vi "Result.Build Attribute Result Item.vi"(6 "ForceFail":bool, 7 "Log(F)/Pass(T)":bool, 8 "Error In(Result Error)":errorcluster, 9 "Value":string, 10 "Name":string, 11 "Category":string) -> (0 "Error Out(No Error)":errorcluster, 2 "Fail/Error":bool, 3 "Attribute":T1 {"Status" items=["LOG", "PASS", "FAIL", "ERROR"]})   [LabVIEW 2018]
uses:
  Result.Attribute.ctl
  Result.Measurement and Attribute Item Status.ctl
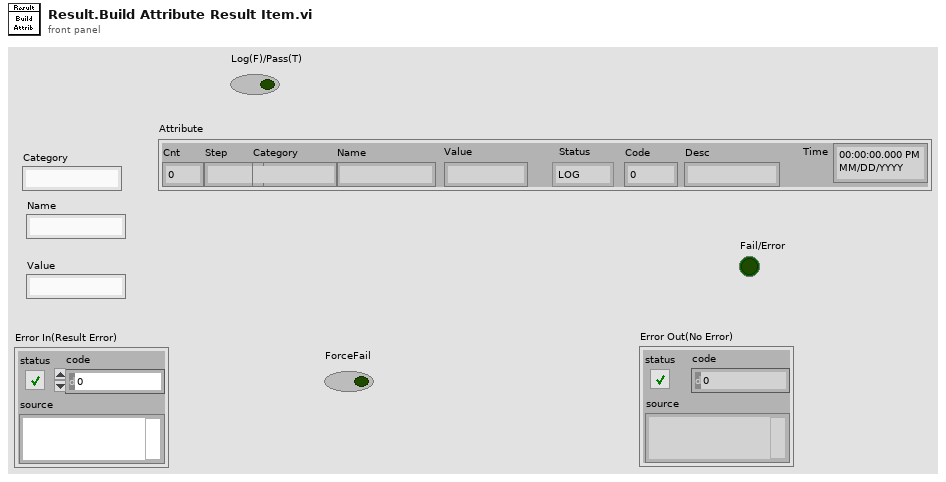
[diagram p1: front panel]
types:
  T1 = typedef "Result.Attribute.ctl" = cluster{"Cnt":i32, "Step":string, "Category":string, "Name":string, "Value":string, "Status":T2, "Code":i32, "Desc":string, "Time":timestamp}
  T2 = typedef "Result.Measurement and Attribute Item Status.ctl" = i32
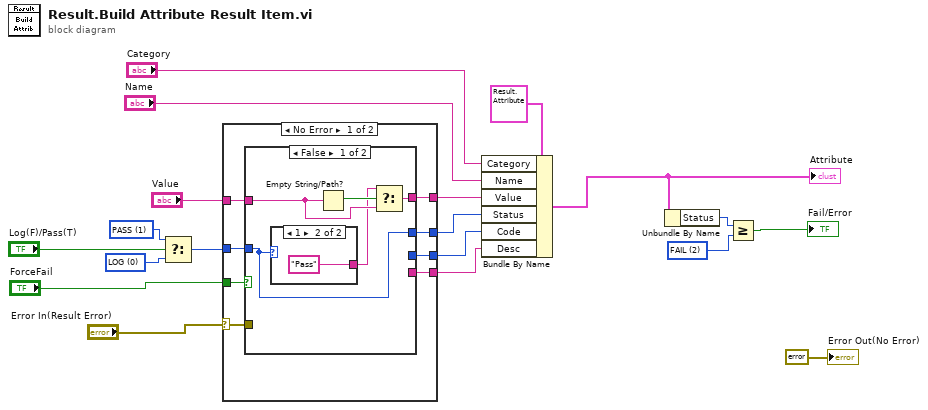
[diagram p0: block diagram]
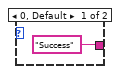
[diagram p2: hidden frame]
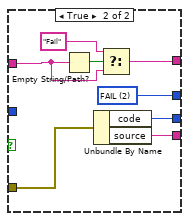
[diagram p3: hidden frame]
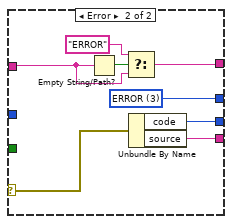
[diagram p4: hidden frame]
diagram:
  w8 = T2 1 items=["LOG", "PASS", "FAIL", "ERROR"] ("Status")
  w7 = T2 0 items=["LOG", "PASS", "FAIL", "ERROR"] ("Status")
  w14 = T2 2 items=["LOG", "PASS", "FAIL", "ERROR"] ("y")
  n1 = Select(t=w8, s="Log(F)/Pass(T)", f=w7) -> (s? t:f=w5:T2)
  n2 = case shown="No Error" "Error In(Result Error)" {
    selector: "Error In(Result Error)" -> [w20 w44]
    tunnel: "ForceFail" -> [w27 _]
    tunnel: [w26 w47] -> w11
    tunnel: [w25 w46] -> w10
    tunnel: [w24 w45] -> w9
    tunnel: w5 -> [w23 _]
    tunnel: "Value" -> [w22 w43]
    tunnel: [w21 w48] -> w2
    frame No Error {
      n3 = case shown="False" w27 {
        tunnel: [w29 w42] -> w26
        tunnel: w20 -> [_ w41]
        tunnel: [_ w40] -> w25
        tunnel: [_ w39] -> w24
        tunnel: w23 -> [w29 _]
        tunnel: w22 -> [w30 w37]
        tunnel: [w31 w35] -> w21
        frame False {
          n4 = case shown="1" w29 {
            tunnel: ["Success" "Pass"] -> w28
            frame 0, Default {
            }
            frame 1 {
            }
          }
          n5 = Empty String/Path?(string/path=w30) -> (empty?=w32:bool)
          n6 = Select(t=w28, s=w32, f=w30) -> (s? t:f=w31:string)
        }
        frame True {
          w42 = T2 2 items=["LOG", "PASS", "FAIL", "ERROR"] ("Status")
          n7 = Empty String/Path?(string/path=w37) -> (empty?=w38:bool)
          n8 = Unbundle By Name(w41) -> ("code"=w40:i32, "source"=w39:string)
          n9 = Select(t="Fail", s=w38, f=w37) -> (s? t:f=w35:string)
        }
      }
    }
    frame Error {
      w47 = T2 3 items=["LOG", "PASS", "FAIL", "ERROR"] ("Status")
      n10 = Empty String/Path?(string/path=w43) -> (empty?=w50:bool)
      n11 = Select(t="ERROR", s=w50, f=w43) -> (s? t:f=w48:string)
      n12 = Unbundle By Name(w44) -> ("code"=w46:i32, "source"=w45:string)
    }
  }
  n13 = Bundle By Name(cluster=T1 {"Cnt"=0, "Step"="", "Category"="", "Name"="", "Value"="", "Status"=0, "Code"=0, "Desc"="", "Time"=timestamp(0 s since 1904-01-01)} ("Attribute"), "Category"="Category", "Name"="Name", "Value"=w2, "Status"=w11, "Code"=w10, "Desc"=w9) -> (w4:T1)
  "Attribute" <- w4
  n14 = Unbundle By Name(w4) -> ("Status"=w15:T2)
  n15 = Greater Or Equal?(x=w15, y=w14) -> (x >= y?=→"Fail/Error":bool)
  "Error Out(No Error)" <- errorcluster {"status"=FALSE, "code"=0, "source"=""} ("Error Out(No Error)")
